vi "Day 9-1.vi"() -> ()   [LabVIEW 2020]
panel:
  out "Numeric":i32
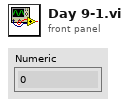
[diagram p1: front panel]
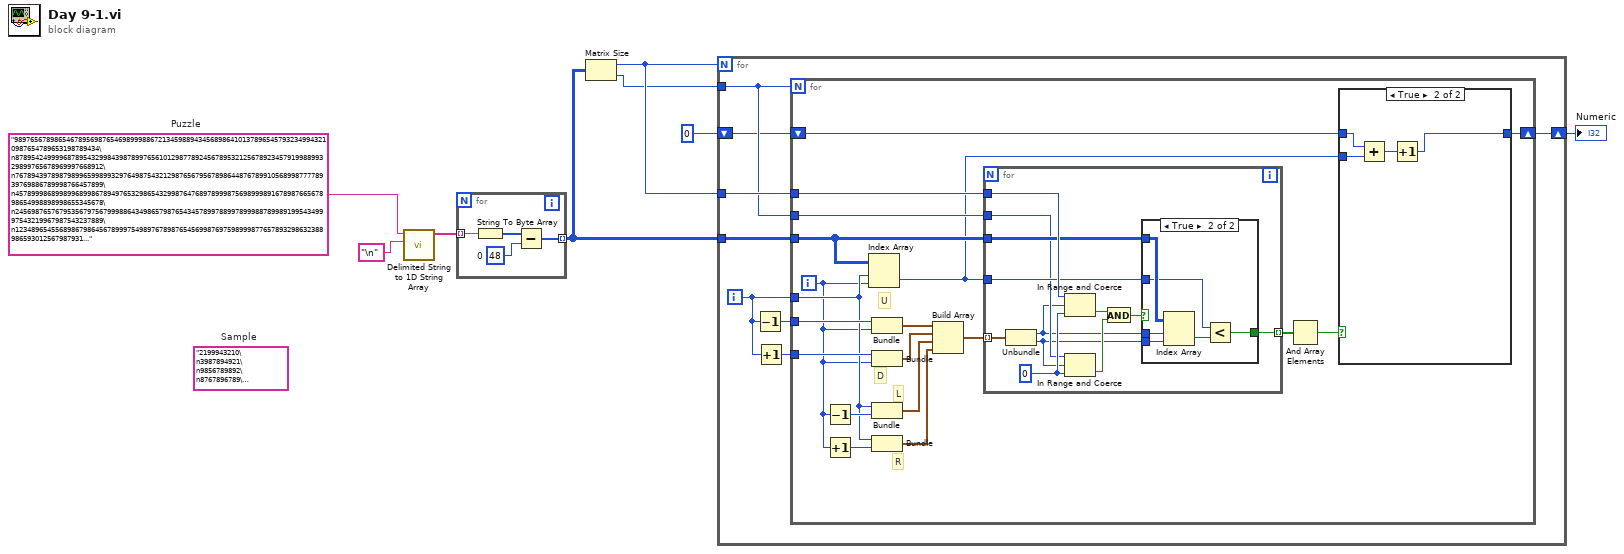
[diagram p0: block diagram]
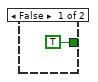
[diagram p3: hidden frame]
diagram:
  (unwired) "2199943210\n3987894921\n9856789892\n8767896789\n9899965678"  # Sample
  w1 = "9897656789865467895698765469899988672134598894345689864101378965457932349943210987654789653198789434\n8789542499996878954329984398789976561012987789245678953212567892345791998899329899765678969997668912\n7678943978987989965998993297649875432129876567956789864487678991056899877778939769886789998766457899\n4578999868998996899867894976532986543299876476897899987569899989167898766567898654998898998655345678\n2456987657679535679756799988643498657987654345789978899789998878998919954349997543219967987543237889\n12348965455689867986456789997549897678987654569987697598999877657893298632388986593012567987931..."  # Puzzle
  n1 = call <vilib>:"Delimited String to 1D String Array.vi"("delimiter"="\n", "delimited string"=w1) -> ("string array"=w7:string[])  [unwired: 9 in]
  n2 = for {
    tunnel: w7 -> [w12] mode=indexing
    tunnel: [w9] -> w6 mode=indexing
    w10 = u8 48  # 0
    n3 = String To Byte Array(string=w12) -> (unsigned byte array=w11:u8[])
    n4 = Subtract(x=w11, y=w10) -> (x-y=w9:u8[])
  }
  n5 = Matrix Size(0:w6) -> (1:w5:i32, 2:w4:i32)
  n6 = for {
    N: w5 -> [_]
    tunnel: w4 -> [w15]
    tunnel: w6 -> [w20]
    tunnel: w5 -> [w16]
    shift-right: [w13] -> w2
    shift-left: 0 -> [w14]
    i -> [w19]
    n7 = Decrement(x=w19) -> (x-1=w18:i32)
    n8 = Increment(x=w19) -> (x+1=w17:i32)
    n9 = for {
      N: w15 -> [_]
      tunnel: w20 -> [w26]
      tunnel: w19 -> [w31]
      tunnel: w18 -> [w39]
      tunnel: w17 -> [w38]
      tunnel: w16 -> [w28]
      tunnel: w15 -> [w27]
      shift-right: [w21] -> w13
      shift-left: w14 -> [w22]
      i -> [w30]
      # "R"
      # "L"
      # "D"
      # "U"
      n10 = Decrement(x=w30) -> (x-1=w37:i32)
      n11 = Increment(x=w30) -> (x+1=w36:i32)
      n12 = Index Array(array=w26, index (row)=w31, index (col)=w30) -> (element=w23:u8)
      n13 = Bundle(w39, w30) -> (w35:cluster{i32, i32})  [unwired: 1 in]
      n14 = Bundle(w38, w30) -> (w34:cluster{i32, i32})  [unwired: 1 in]
      n15 = Bundle(w31, w37) -> (w33:cluster{i32, i32})  [unwired: 1 in]
      n16 = Bundle(w31, w36) -> (w32:cluster{i32, i32})  [unwired: 1 in]
      n17 = Build Array(w35, w34, w33, w32) -> (w29:cluster{i32, i32}[])
      n18 = for {
        tunnel: w29 -> [w56] mode=indexing
        tunnel: w28 -> [w55]
        tunnel: w27 -> [w48]
        tunnel: w23 -> [w51]
        tunnel: w26 -> [w50]
        tunnel: [w45] -> w25 mode=indexing
        w54 = 0 ("lower limit")
        n19 = Unbundle(w56) -> (w47:i32, w46:i32)
        n20 = In Range and Coerce(upper limit=w55, x=w47, lower limit=w54) -> (In Range?=w53:bool)  [unwired: 1 out]
        n21 = In Range and Coerce(upper limit=w48, x=w46, lower limit=w54) -> (In Range?=w52:bool)  [unwired: 1 out]
        n22 = And(x=w53, y=w52) -> (x .and. y?=w49:bool)
        n23 = case shown="True" w49 {
          tunnel: w51 -> [_ w60]
          tunnel: w50 -> [_ w63]
          tunnel: w47 -> [_ w62]
          tunnel: w46 -> [_ w61]
          tunnel: [TRUE w58] -> w45
          frame False {
          }
          frame True {
            n24 = Index Array(array=w63, index (row)=w62, index (col)=w61) -> (element=w59:u8)
            n25 = Less?(x=w60, y=w59) -> (x < y?=w58:bool)
          }
        }
      }
      n26 = And Array Elements(Boolean array=w25) -> (logical AND=w24:bool)
      n27 = case shown="True" w24 {
        tunnel: w23 -> [_ w44]
        tunnel: w22 -> [w40 w43]
        tunnel: [w40 w41] -> w21
        frame False {
        }
        frame True {
          n28 = Add(x=w43, y=w44) -> (x+y=w42:i32)
          n29 = Increment(x=w42) -> (x+1=w41:i32)
        }
      }
    }
  }
  "Numeric" <- w2
